vi "Extract Segment.vi"(6 "Containing Type":T2, 8 "error in (no error)":errorcluster, 9 "In Type":bool, 10 "String":string, 11 "ProtoParser in":refnum<class "ProtoParser.lvclass">) -> (0 "error out":errorcluster, 1 "Segment":T1, 2 "Remaining":string, 3 "ProtoParser out":refnum<class "ProtoParser.lvclass">)   [LabVIEW 2020, in "LV-Protoc.lvlib" / "ProtoParser.lvclass"]
uses:
  ProtoParser.lvclass
  Segment Type.ctl
  Raw Segment.ctl
  LV-Protoc.lvlib
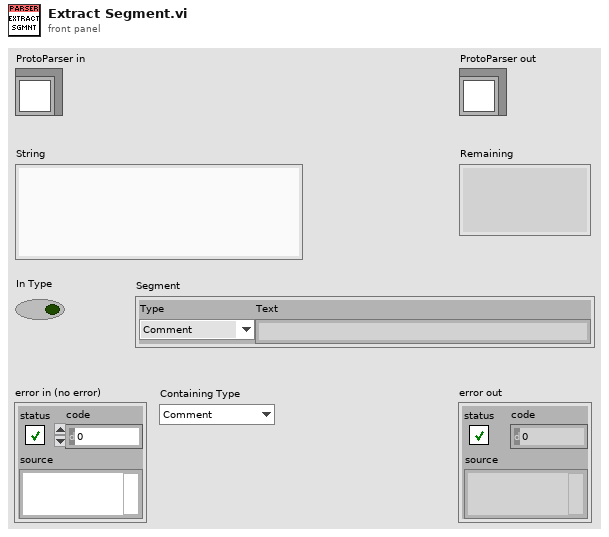
[diagram p1: front panel]
types:
  T1 = typedef "LV-Protoc.lvlib/Raw Segment.ctl" = cluster{"Type":T2, "Text":string}
  T2 = typedef "LV-Protoc.lvlib/Segment Type.ctl" = enum16{"Comment", "Message Open", "Enum Open", "Message Close", "Enum Close", "Field", "Syntax", "Import", "Enum Value", "Package", "Reserved"}
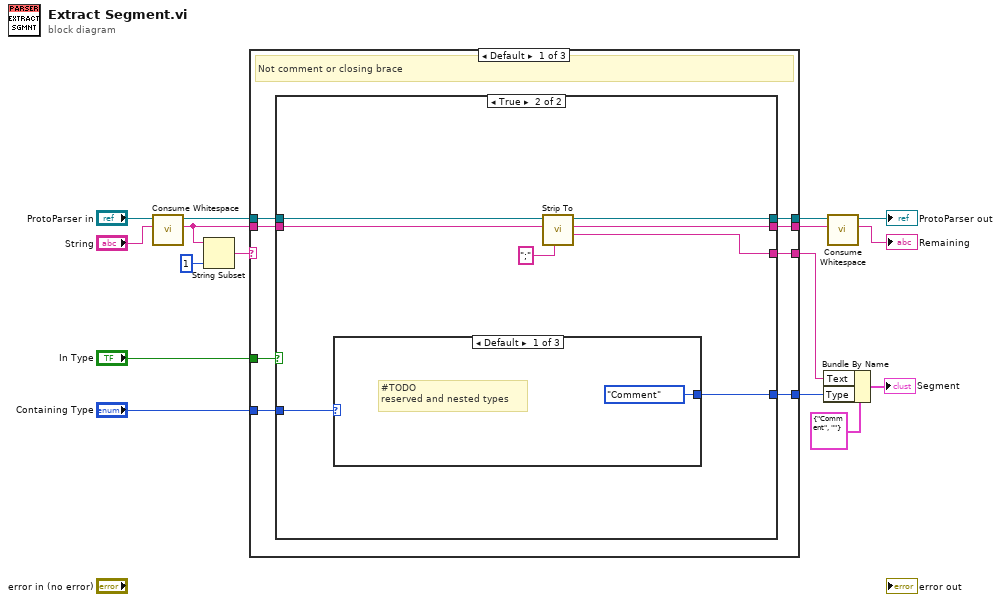
[diagram p0: block diagram]
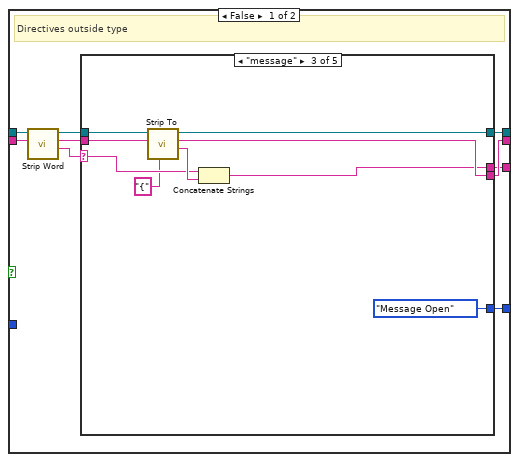
[diagram p2: hidden frame]
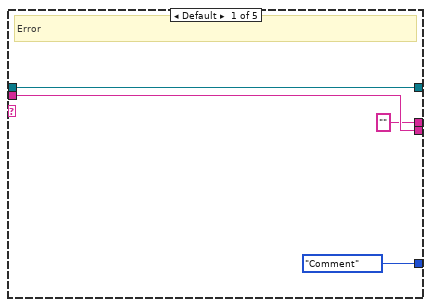
[diagram p3: hidden frame]
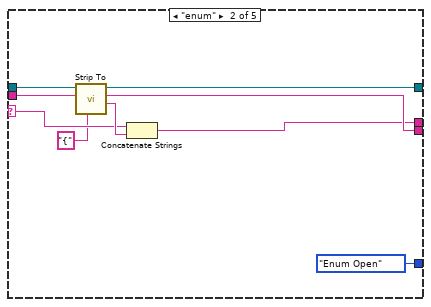
[diagram p4: hidden frame]
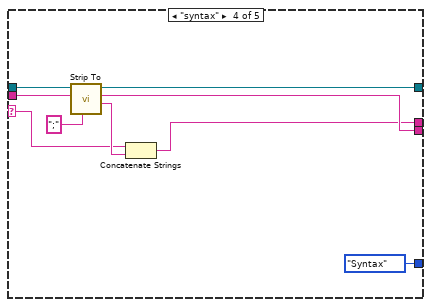
[diagram p5: hidden frame]
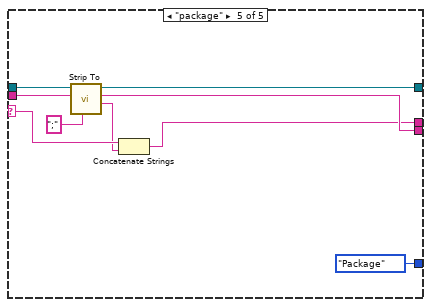
[diagram p6: hidden frame]
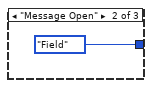
[diagram p7: hidden frame]
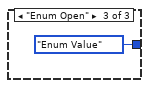
[diagram p8: hidden frame]
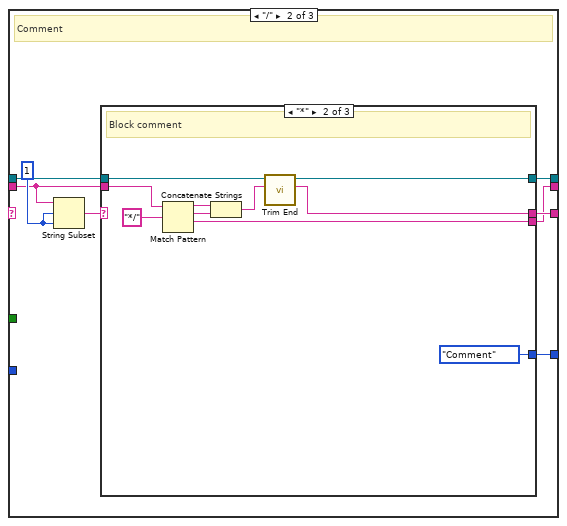
[diagram p9: hidden frame]
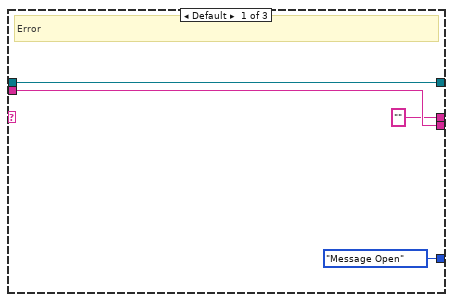
[diagram p10: hidden frame]
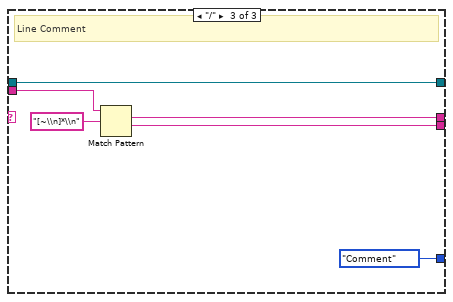
[diagram p11: hidden frame]
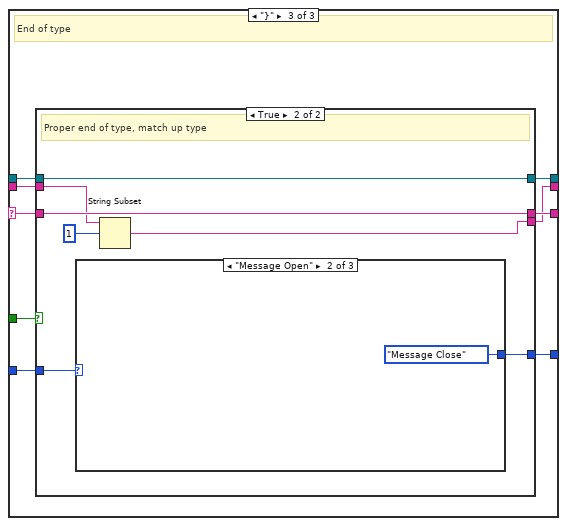
[diagram p12: hidden frame]
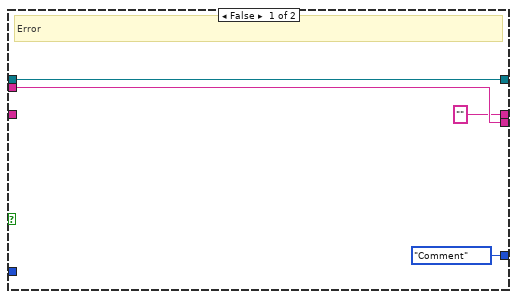
[diagram p13: hidden frame]
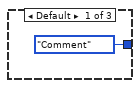
[diagram p14: hidden frame]
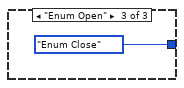
[diagram p15: hidden frame]
diagram:
  n1 = call "Consume Whitespace.vi"("String"="String", "ProtoParser in"="ProtoParser in") -> ("Remaining"=w11:string, "ProtoParser out"=w10:refnum<class "ProtoParser.lvclass">)  [unwired: 7 in, 1 out]
  n2 = String Subset(string=w11, length (rest)=1 ("length (rest)")) -> (substring=w13:string)  [unwired: 1 in]
  n3 = case shown="Default" w13 {
    selector: w13 -> [_ _ w116]
    tunnel: "In Type" -> [w24 _ w119]
    tunnel: w11 -> [w22 w90 w120]
    tunnel: [w18 w89 w115] -> w5
    tunnel: [w17 w88 w117] -> w6
    tunnel: [w19 w87 w113] -> w2
    tunnel: w10 -> [w23 w86 w121]
    tunnel: [w20 w85 w114] -> w4
    tunnel: "Containing Type" -> [w21 _ w118]
    frame Default {
      # "Not comment or closing brace"
      n4 = case shown="True" w24 {
        tunnel: w23 -> [w33 w77]
        tunnel: w22 -> [w32 w76]
        tunnel: w21 -> [_ w75]
        tunnel: [w28 w81] -> w20
        tunnel: [w27 w80] -> w19
        tunnel: [w26 w78] -> w18
        tunnel: [w25 w74] -> w17
        frame False {
          # "Directives outside type"
          n5 = call "Strip Word.vi"("String"=w32, "ProtoParser in"=w33) -> ("Word"=w29:string, "Remaining"=w30:string, "ProtoParser out"=w31:refnum<class "ProtoParser.lvclass">)  [unwired: 6 in, 1 out]
          n6 = case shown="\"message\"" w29 {
            selector: w29 -> [_ w41 w50 w57 w67]
            tunnel: w31 -> [w37 w46 w55 w64 w73]
            tunnel: w30 -> [w36 w44 w53 w63 w72]
            tunnel: [w37 w45 w54 w61 w70] -> w28
            tunnel: [w36 w43 w52 w62 w71] -> w27
            tunnel: ["" w40 w49 w56 w65] -> w26
            tunnel: [Segment_Type."Comment" ("Type") Segment_Type."Enum Open" ("Type") Segment_Type."Message Open" ("Type") Segment_Type."Syntax" ("Type") Segment_Type."Package" ("Type")] -> w25
            frame Default {
              # "Error"
            }
            frame "enum" {
              n7 = call "Strip To.vi"("End"="{", "String"=w44, "ProtoParser in"=w46) -> ("Portion"=w42:string, "Remaining"=w43:string, "ProtoParser out"=w45:refnum<class "ProtoParser.lvclass">)  [unwired: 5 in, 1 out]
              n8 = Concatenate Strings(w41, w42) -> (w40:string)
            }
            frame "message" {
              n9 = call "Strip To.vi"("End"="{", "String"=w53, "ProtoParser in"=w55) -> ("Portion"=w51:string, "Remaining"=w52:string, "ProtoParser out"=w54:refnum<class "ProtoParser.lvclass">)  [unwired: 5 in, 1 out]
              n10 = Concatenate Strings(w50, w51) -> (w49:string)
            }
            frame "syntax" {
              n11 = call "Strip To.vi"("End"=";", "String"=w63, "ProtoParser in"=w64) -> ("Portion"=w58:string, "Remaining"=w62:string, "ProtoParser out"=w61:refnum<class "ProtoParser.lvclass">)  [unwired: 5 in, 1 out]
              n12 = Concatenate Strings(w57, w58) -> (w56:string)
            }
            frame "package" {
              n13 = call "Strip To.vi"("End"=";", "String"=w72, "ProtoParser in"=w73) -> ("Portion"=w66:string, "Remaining"=w71:string, "ProtoParser out"=w70:refnum<class "ProtoParser.lvclass">)  [unwired: 5 in, 1 out]
              n14 = Concatenate Strings(w67, w66) -> (w65:string)
            }
          }
        }
        frame True {
          n15 = case shown="Default" w75 {
            tunnel: [Segment_Type."Comment" ("Type") Segment_Type."Field" ("Type") Segment_Type."Enum Value" ("Type")] -> w74
            frame Default {
              # "#TODO\nreserved and nested types"
            }
            frame "Message Open" {
            }
            frame "Enum Open" {
            }
          }
          n16 = call "Strip To.vi"("End"=";", "String"=w76, "ProtoParser in"=w77) -> ("Portion"=w78:string, "Remaining"=w80:string, "ProtoParser out"=w81:refnum<class "ProtoParser.lvclass">)  [unwired: 5 in, 1 out]
        }
      }
    }
    frame "/" {
      w92 = 1 ("offset (0)")
      # "Comment"
      n17 = String Subset(string=w90, offset (0)=w92, length (rest)=w92) -> (substring=w91:string)
      n18 = case shown="\"*\"" w91 {
        tunnel: w90 -> [w94 w105 w112]
        tunnel: ["" ("Remaining") w97 w110] -> w89
        tunnel: [Segment_Type."Message Open" ("Type") Segment_Type."Comment" ("Type") Segment_Type."Comment" ("Type")] -> w88
        tunnel: [w94 w103 w108] -> w87
        tunnel: w86 -> [w96 w106 w107]
        tunnel: [w96 w99 w107] -> w85
        frame Default {
          # "Error"
        }
        frame "*" {
          # "Block comment"
          n19 = Match Pattern(string=w105, regular expression="*/") -> (before substring=w102:string, match substring=w101:string, after substring=w103:string)  [unwired: 1 in, 1 out]
          n20 = Concatenate Strings(w102, w101) -> (w98:string)
          n21 = call "Trim End.vi"("String"=w98, "ProtoParser in"=w106) -> ("Trimmed"=w97:string, "ProtoParser out"=w99:refnum<class "ProtoParser.lvclass">)  [unwired: 7 in, 1 out]
        }
        frame "/" {
          # "Line Comment"
          n22 = Match Pattern(string=w112, regular expression="[~\\n]*\\n") -> (match substring=w110:string, after substring=w108:string)  [unwired: 1 in, 2 out]
        }
      }
    }
    frame "}" {
      # "End of type"
      n23 = case shown="True" w119 {
        tunnel: w121 -> [w125 w129]
        tunnel: w120 -> [w124 w128]
        tunnel: w118 -> [_ w132]
        tunnel: [Segment_Type."Comment" ("Type") w131] -> w117
        tunnel: w116 -> [_ w130]
        tunnel: ["" w130] -> w115
        tunnel: [w125 w129] -> w114
        tunnel: [w124 w126] -> w113
        frame False {
          # "Error"
        }
        frame True {
          # "Proper end of type, match up type"
          n24 = case shown="\"Message Open\"" w132 {
            tunnel: [Segment_Type."Comment" ("Type") Segment_Type."Message Close" ("Type") Segment_Type."Enum Close" ("Type")] -> w131
            frame Default {
            }
            frame "Message Open" {
            }
            frame "Enum Open" {
            }
          }
          n25 = String Subset(string=w128, offset (0)=1) -> (substring=w126:string)  [unwired: 1 in]
        }
      }
    }
  }
  n26 = Bundle By Name(cluster=T1 {"Type"=enum."Comment", "Text"=""} ("Segment"), "Text"=w5, "Type"=w6) -> (→"Segment":T1)
  n27 = call "Consume Whitespace.vi"("String"=w2, "ProtoParser in"=w4) -> ("Remaining"=→"Remaining":string, "ProtoParser out"=→"ProtoParser out":refnum<class "ProtoParser.lvclass">)  [unwired: 7 in, 1 out]
